vi "thread.vi"(0 "HGF_TimeoutWorker":refnum<class "HGF_TimeoutWorker.lvclass">, 1 "HGF_ThreadPool_Reference":refnum<class "HGF_Reference.lvclass">, 5 "error in (no error)":errorcluster) -> (19 "error out":errorcluster)   [LabVIEW 2014, in "HGF_BaseClasses.lvlib" / "HGF_TimeoutWorker.lvclass"]
doc: "This is the thread started from the HGF_ThreadPool.\n\n<b>Attention:</b> This VI is reentrant and sharing sources."
uses:
  HGF_TimeoutWorker.lvclass
  HGF_Auxiliary/HGF_Auxiliary.lvlib
  HGF_BaseClasses/HGF_ThreadTask/HGF_ThreadTask.lvclass
  HGF_BaseClasses/HGF_Event/HGF_Event.lvclass
  HGF_BaseClasses/HGF_ThreadPool/HGF_ThreadPool.lvclass
  HGF_BaseClasses/HGF_Reference/HGF_Reference.lvclass
  HGF_BaseClasses/HGF_ThreadWorker/HGF_ThreadWorker.lvclass
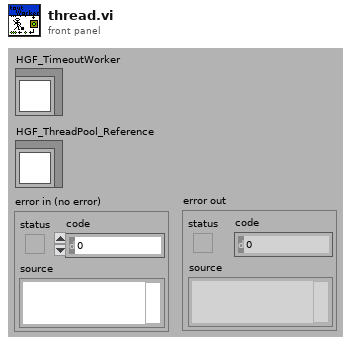
[diagram p1: front panel]
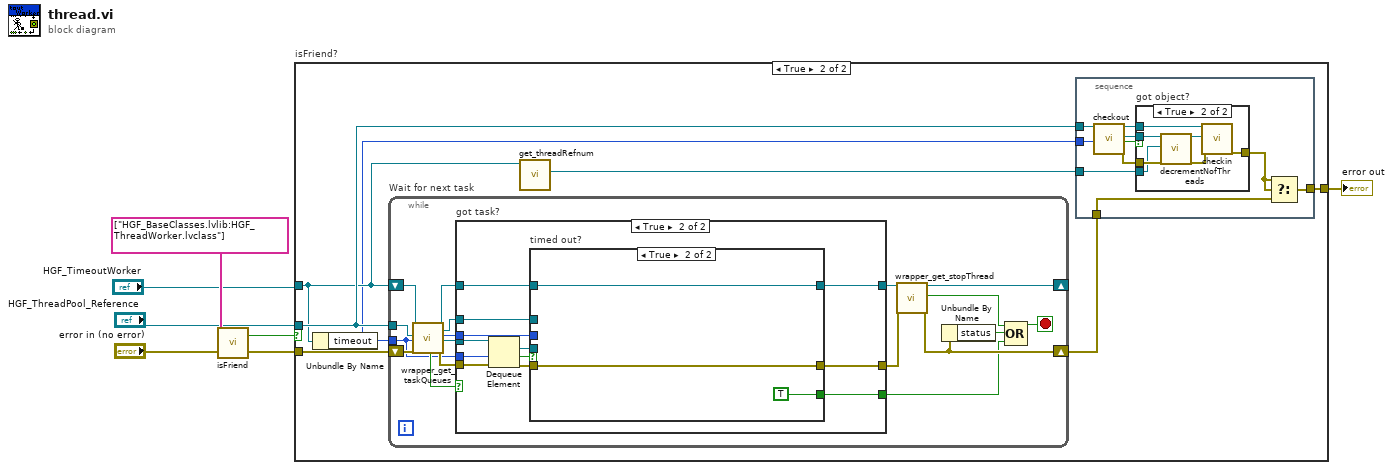
[diagram p0: block diagram]
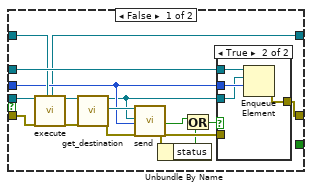
[diagram p5: hidden frame]
diagram:
  n1 = call "isFriend.vi"("error in (no error)"="error in (no error)", "Friends"=string[] ["HGF_BaseClasses.lvlib:HGF_ThreadWorker.lvclass"]) -> ("error out"=w5:errorcluster, "isFriend?"=w7:bool)
  n2 = case "isFriend?" shown="True" w7 {
    tunnel: "HGF_ThreadPool_Reference" -> [_ w15]
    tunnel: [w8 w13] -> w1
    tunnel: "HGF_TimeoutWorker" -> [_ w10]
    tunnel: w5 -> [w8 w12]
    frame False {
    }
    frame True {
      n3 = Unbundle By Name(w10) -> ("timeout"=w9:i32)
      n4 = while "Wait for next task" {
        shift-right: [w48] -> _
        shift-left: w10 -> [w44]
        tunnel: w15 -> [w36]
        shift-right: [w46] -> w14
        shift-left: w12 -> [w42]
        tunnel: w9 -> [w34]
        stop <- w51 stop-if-true
        n5 = call "wrapper_get_taskQueues.vi"("HGF_ThreadWorker in"=w44, "HGF_ThreadPool_Reference"=w36, "timeout in ms (-1)"=w34, "error in (no error)"=w42) -> ("got object?"=w40:bool, "HGF_ThreadWorker in"=w43:refnum<class "HGF_ThreadWorker.lvclass">, "taskQueue out"=w39:refnum<queue>, "timeoutTaskQueueOut"=w38:i32, "taskQueue in"=w37:refnum<queue>, "error out"=w41:errorcluster)  [unwired: 9 in, 1 out]
        n6 = case "got task?" shown="True" w40 {
          tunnel: w41 -> [w53 w65]
          tunnel: w39 -> [_ w64]
          tunnel: w37 -> [_ w63]
          tunnel: w43 -> [w52 w60]
          tunnel: w38 -> [_ w62]
          tunnel: [w53 w61] -> w45
          tunnel: [w52 w56] -> w49
          tunnel: [_ w55] -> w35
          tunnel: w34 -> [_ w54]
          frame False {
          }
          frame True {
            n7 = Dequeue Element(queue=w63, timeout in ms (-1)=w54, error in (no error)=w65) -> (element=w59:refnum<class "HGF_ThreadTask.lvclass">, timed out?=w57:bool, error out=w58:errorcluster)  [unwired: 1 out]
            n8 = case "timed out?" shown="True" w57 {
              tunnel: w64 -> [w81 _]
              tunnel: w62 -> [w72 _]
              tunnel: [w66 w89] -> w56
              tunnel: [w80 w88] -> w61
              tunnel: w60 -> [w77 w89]
              tunnel: w59 -> [w79 _]
              tunnel: w58 -> [w78 w88]
              tunnel: [_ TRUE] -> w55
              frame False {
                n9 = call "execute.vi"("HGF_ThreadTask"=w79, "error in (no error)"=w78, "HGF_ThreadWorker"=w77) -> ("dup HGF_ThreadWorker"=w66:refnum<class "HGF_ThreadWorker.lvclass">, "HGF_ThreadTask"=w76:refnum<class "HGF_ThreadTask.lvclass">, "error out"=w75:errorcluster)  [unwired: 14 out]
                n10 = call "get_destination.vi"("HGF_ThreadTask"=w76, "error in (no error)"=w75) -> ("dup HGF_ThreadTask"=w71:refnum<class "HGF_ThreadTask.lvclass">, "destination"=w74:refnum<class "HGF_Event.lvclass">, "error out"=w73:errorcluster)  [unwired: 15 out]
                n11 = call-dynamic "send.vi"("HGF_Event"=w74, "Object"=w71, "timeout in ms (-1)"=w72, "error in (no error)"=w73) -> ("timed out?"=w69:bool, "error out"=w68:errorcluster)  [unwired: 1 in, 13 out]
                n12 = Unbundle By Name(w68) -> ("status"=w67:bool)
                n13 = Or(x=w69, y=w67) -> (x .or. y?=w70:bool)
                n14 = case shown="True" w70 {
                  tunnel: w81 -> [_ w86]
                  tunnel: [w82 w85] -> w80
                  tunnel: w72 -> [_ w84]
                  tunnel: w71 -> [_ w83]
                  tunnel: w68 -> [w82 _]
                  frame False {
                  }
                  frame True {
                    n15 = Enqueue Element(queue=w86, element=w83, timeout in ms (-1)=w84) -> (error out=w85:errorcluster)  [unwired: 1 in, 2 out]
                  }
                }
              }
              frame True {
              }
            }
          }
        }
        n16 = call-dynamic "wrapper_get_stopThread.vi"("HGF_ThreadWorker in"=w49, "error in (no error)"=w45) -> ("HGF_ThreadWorker out"=w48:refnum<class "HGF_ThreadWorker.lvclass">, "stopThread"=w47:bool, "error out"=w46:errorcluster)  [unwired: 15 in]
        n17 = Unbundle By Name(w46) -> ("status"=w50:bool)
        n18 = Compound Arithmetic op=OR(w47, w50, w35) -> (w51:bool)
      }
      n19 = call "get_threadRefnum.vi"("HGF_ThreadWorker in"=w10) -> ("threadRefnum"=w11:refnum<vi>)  [unwired: 8 in, 2 out]
      n20 = stacked-sequence {
        tunnel: w15 -> [w25]
        tunnel: w14 -> [w19]
        tunnel: w9 -> [w24]
        tunnel: [w18] -> w13
        tunnel: w11 -> [w16]
        frame #0 {
          n21 = call "checkout.vi"("HGF_ThreadPool_Reference"=w25, "timeout in ms (-1)"=w24) -> ("dup HGF_ThreadPool_Reference"=w21:refnum<class "HGF_Reference.lvclass">, "HGF_ThreadPool"=w23:refnum<class "HGF_ThreadPool.lvclass">, "got object?"=w20:bool, "error out"=w22:errorcluster)  [unwired: 1 in, 13 out]
          n22 = case "got object?" shown="True" w20 {
            tunnel: w23 -> [_ w33]
            tunnel: w22 -> [w26 w32]
            tunnel: w21 -> [_ w31]
            tunnel: [w26 w28] -> w17
            tunnel: w16 -> [_ w27]
            frame False {
            }
            frame True {
              n23 = call "decrementNofThreads.vi"("HGF_ThreadPool"=w33, "threadRef"=w27, "error in (no error)"=w32) -> ("dup HGF_ThreadPool"=w30:refnum<class "HGF_ThreadPool.lvclass">, "error out"=w29:errorcluster)  [unwired: 15 out]
              n24 = call "checkin.vi"("HGF_Reference"=w31, "Object"=w30, "error in (no error)"=w29) -> ("error out"=w28:errorcluster)  [unwired: 1 in, 15 out]
            }
          }
          n25 = Select(t=w17, s=w17, f=w19) -> (s? t:f=w18:errorcluster)
        }
      }
    }
  }
  "error out" <- w1
